vi "Listen.vi"(8 "error in":errorcluster) -> (0 "error out":errorcluster)   [LabVIEW 2016, in "TCP.lvlib"]
uses:
  Support/Message Queue/Enqueue Message (Single).vi
  TCP.lvlib
  support/Message Queue/Message Queue.lvlib
panel:
  in  "Action":enum16{"GET", "SET"}(ring)
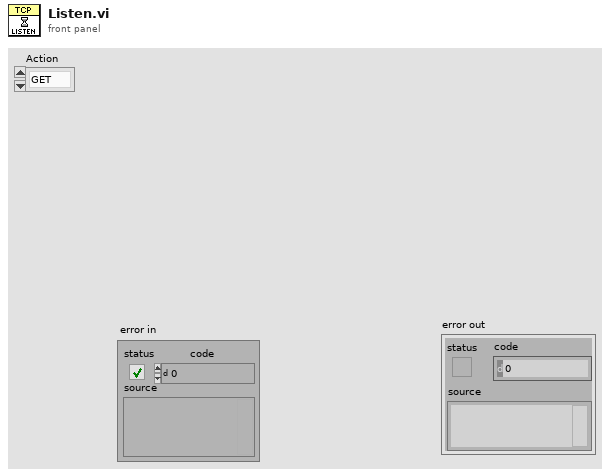
[diagram p1: front panel]
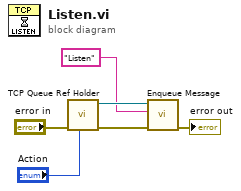
[diagram p0: block diagram]
diagram:
  n1 = call "TCP Queue Ref Holder.vi"("Action"="Action", "error in"="error in") -> ("error out"=w5:errorcluster, "Input Message Queue"=w3:refnum<queue>)  [unwired: 8 in]
  n2 = call-poly "Enqueue Message.vi"("error in (no error)"=w5, "Message"="Listen", "Message Queue"=w3) -> ("error out"=→"error out":errorcluster)  [unwired: 7 in, 1 out]
